vi "调用节点.vi"() -> ()   [LabVIEW 2018]
panel:
  in  "数值":dbl=5.0
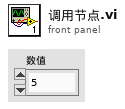
[diagram p1: front panel]
types:
  T1 = enum32{"Invalid", "Standard", "Closed", "Hidden", "Minimized", "Maximized"}
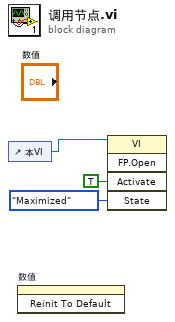
[diagram p0: block diagram]
diagram:
  n1 = control-ref of="本VI"() -> (w3:refnum<vi>)
  n2 = invoke on="数值" class="DigNum (严格)" method="Reinit To Default"() -> ()  [unwired: 3 in, 3 out]
  n3 = invoke class="VI" method="FP.Open"(reference=w3, "Activate"=TRUE ("激活？"), "State"=T1."Maximized" ("状态")) -> ()  [unwired: 2 in, 5 out]
